vi "000_Project Manage.vi"(11 "Queue Ref In":T1={"UI"=refnum, "Message"=refnum, "Data"=refnum, "Caller"=refnum, "Name"="000 Common", "Data Path"=path "", "Class Path"=path "", "SubPanel"=refnum, "Project Name"="", "MNT"="", "Title"="", "Data Source"=refnum, "Queue List"={}, "VI"=refnum, "UE"=refnum}) -> ()   [LabVIEW 2020]
doc: "PM"
uses:
  Alin/QMH/000 Module Data Type.ctl
  Alin/QMH/Queue Message.ctl
  9999 SubVI/Global/Data Global/Data Global Mode.ctl
  ed3733e6-0b6c-4e46-af2e-562a3ca12228.vi
  <vilib>/Utility/file.llb/Read Delimited Spreadsheet (string).vi
  006 Path Management/006 System Gloabl.vi
  <vilib>/zip/NI_Unzip.lvlib
panel:
  in  "Project Refresh":bool
  in  "Monitor":bool
  in  "Project Set":bool
  in  "Project Copy":bool
  in  "Project Export":bool
  in  "Project Import":bool
  in  "Project Launch":bool
  in  "Project Delete":bool
  in  "Project List":i32(listbox)
  in  "Panel Hidden":bool
  in  "Data Source List":string(tree)
  out "Count":string
  in  "Device List":i32(listbox)
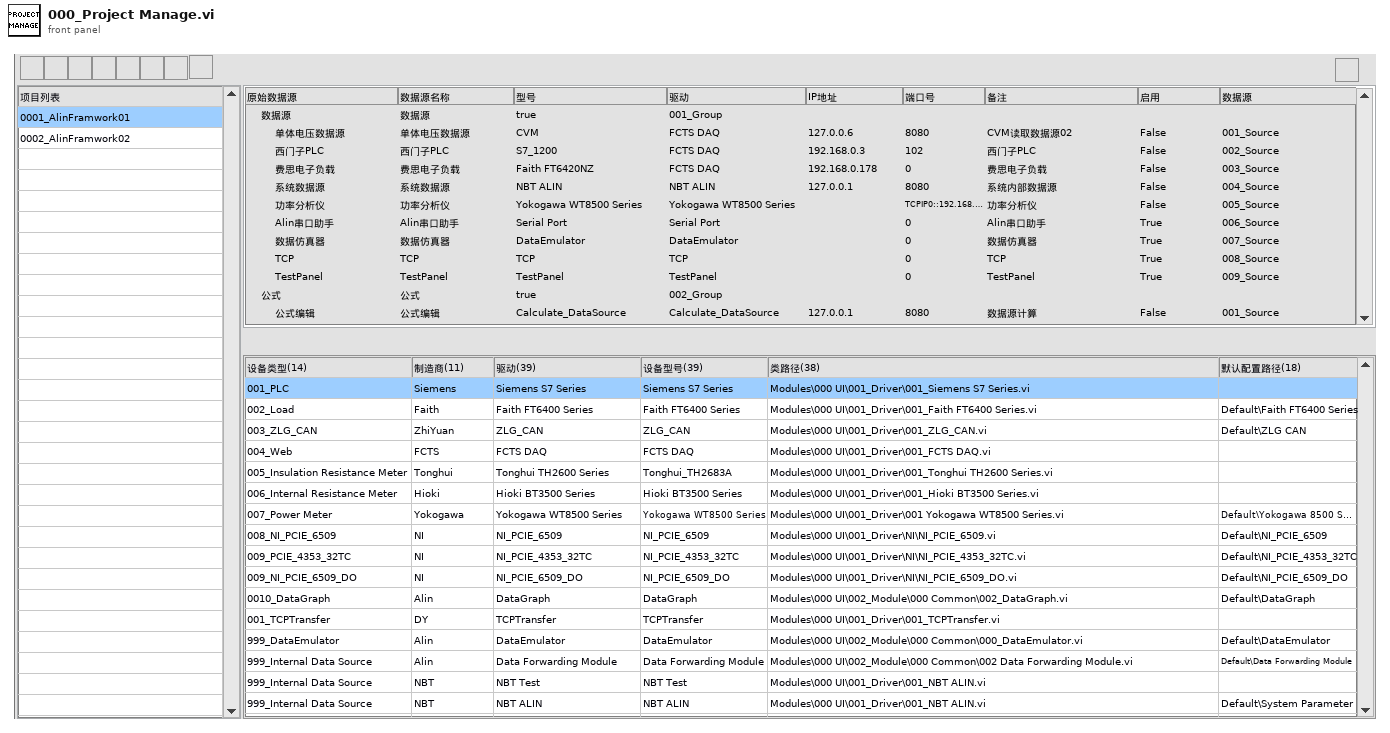
[diagram p1: front panel]
types:
  T1 = typedef "000 Module Data Type.ctl" = cluster{"UI":refnum<queue>, "Message":refnum<queue>, "Data":refnum<queue>, "Caller":refnum<queue>, "Name":string, "Data Path":path, "Class Path":path, "SubPanel":refnum<vi>, "Project Name":string, "MNT":string, "Title":string, "Data Source":refnum<queue>, "Queue List":map{string, refnum<queue>}, "VI":refnum<vi>, "UE":refnum<user-event>}
  T2 = cluster{"Project":string, "Queue List":map{string, refnum<queue>}, "Queue Ref":T1, "RootPath":path, "Device List Ref":refnum<vi>, "Config Path":path, "Project List Value":i32, "Project List":string[], "Project List Refer":refnum<vi>, "Source":refnum<vi>, "Source Path":path}
  T3 = cluster{"Read Data":map{string, string}, "Send Data":map{string, string}, "Open?":bool, "Start?":bool, "Queue Ref":T1, "Device List":refnum<vi>}
  T4 = enum32{"Invalid", "Standard", "Closed", "Hidden", "Minimized", "Maximized"}
  T5 = typedef "eventvkey.ctl" = enum16{"ASCII", "Enter", "Return", "Shift", "Ctrl", "Alt", "Cmd", "Opt", "Caps", "NumLock", "Clear", "Break", "Up", "Down", "Left", "Right", "Insert", "Delete", "Home", "End", "PageUp", "PageDown", "Escape", "Help", "Pause", "ScrollLock", "F1", "F2", "F3", "F4", "F5", "F6", "F7", "F8", "F9", "F10", "F11", "F12", "F13", "F14", "F15", "F16", "F17", "F18", "F19", "F20", "F21", "F22", "F23", "F24", "Play", "VolumeUp", "VolumeDown", "Mute", "Two Byte Char"}
  T6 = cluster{"Shift":bool, "Ctrl":bool, "Alt":bool, "Cmd":bool, "Opt":bool}
  T7 = typedef "Data Global Mode.ctl" = enum16{"Init", "Read", "Write", "Write Data", "Load"}
  T8 = enum32{"invalid app kind", "Development System", "Run Time System", "Student Edition", "Embedded LabVIEW", "Evaluation", "Custom"}
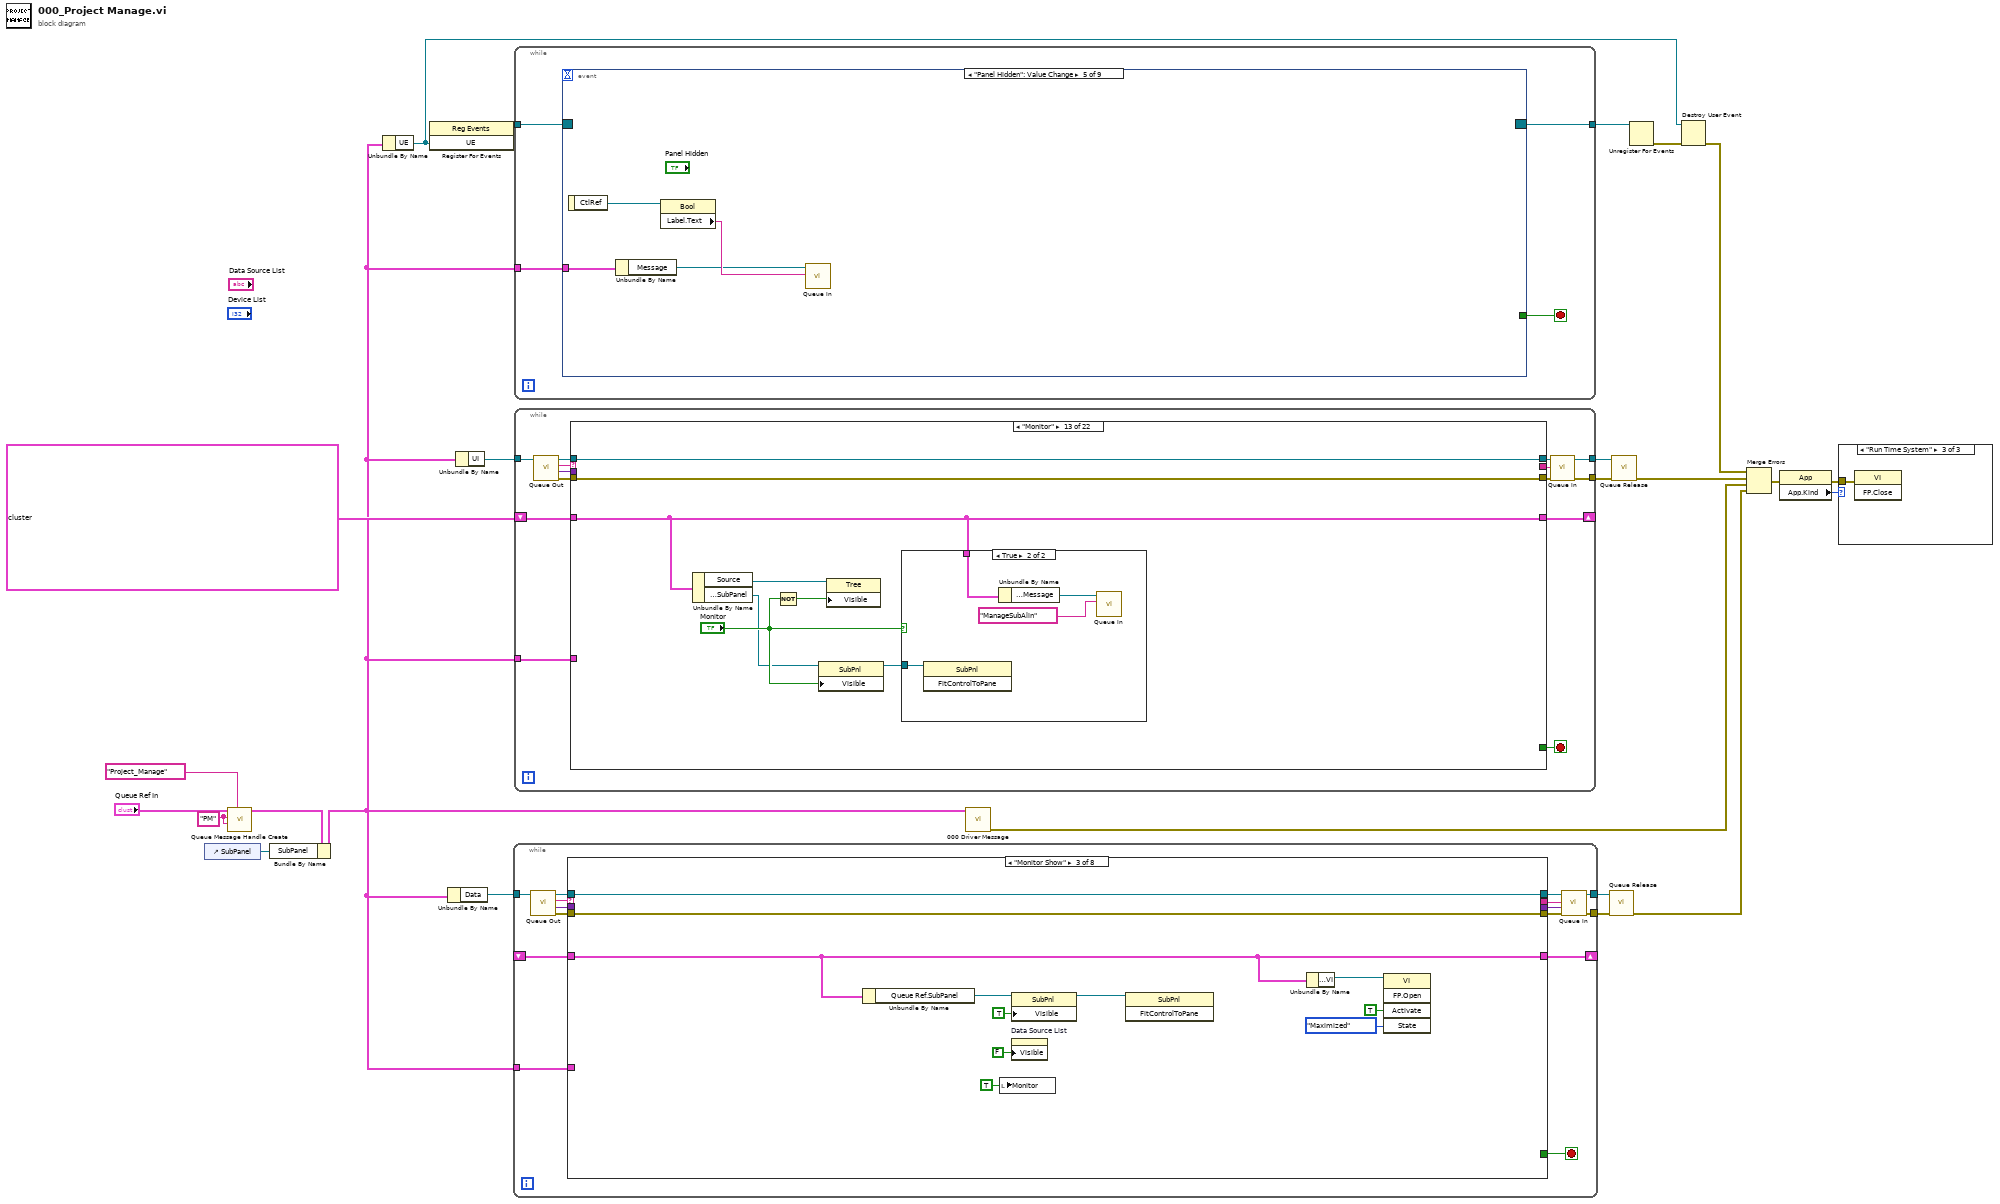
[diagram p0: block diagram]
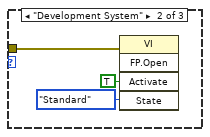
[diagram p3: hidden frame]
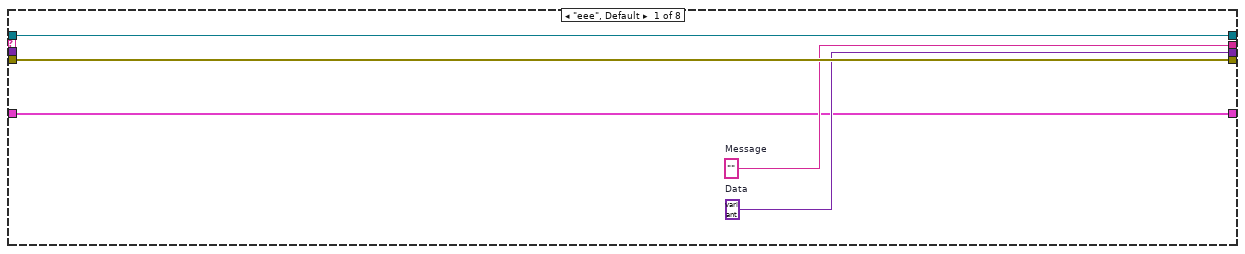
[diagram p4: hidden frame]
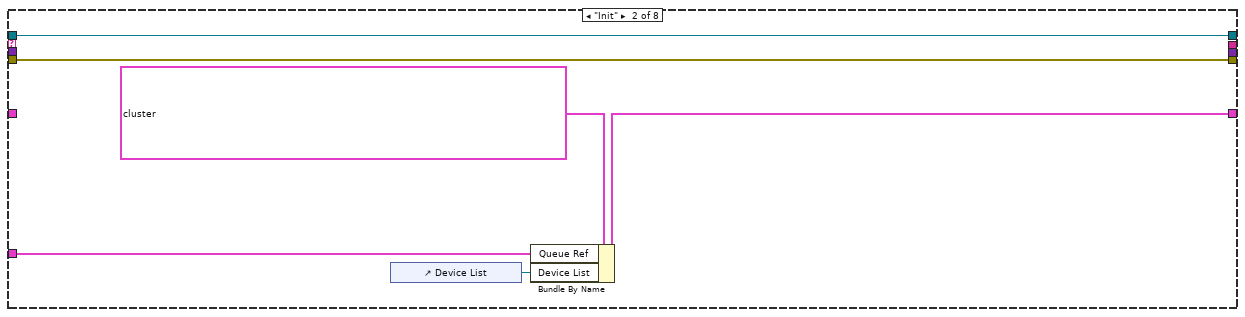
[diagram p5: hidden frame]
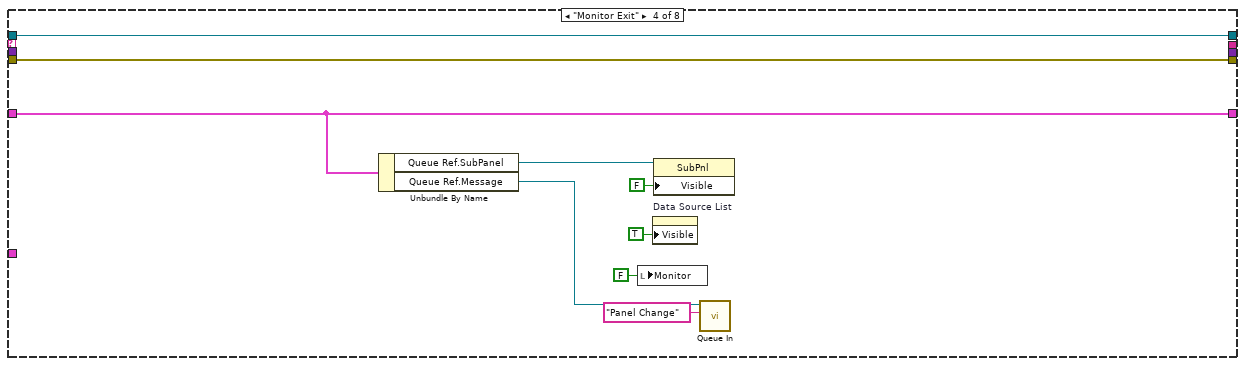
[diagram p6: hidden frame]
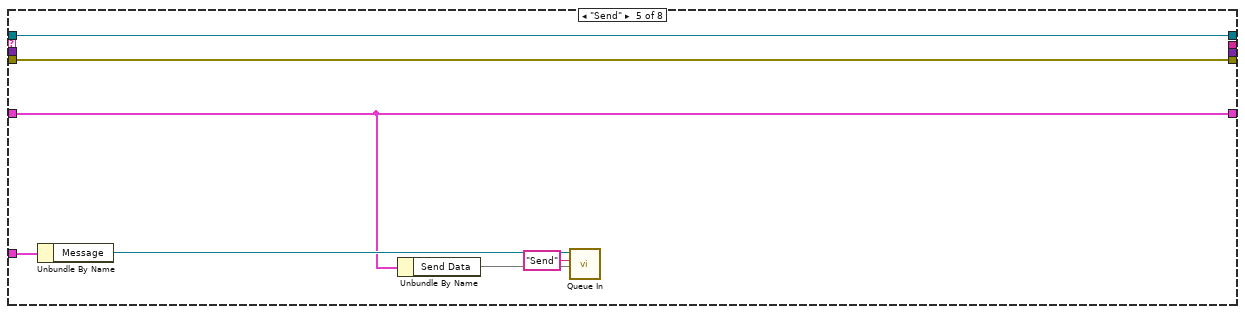
[diagram p7: hidden frame]
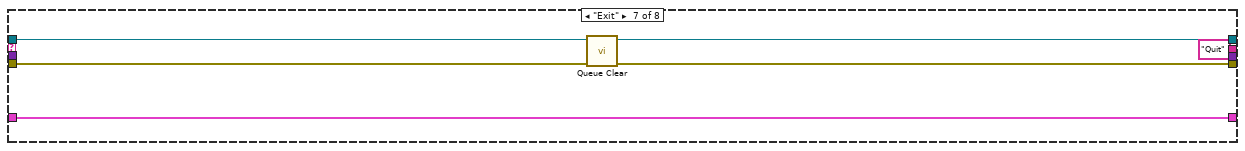
[diagram p9: hidden frame]
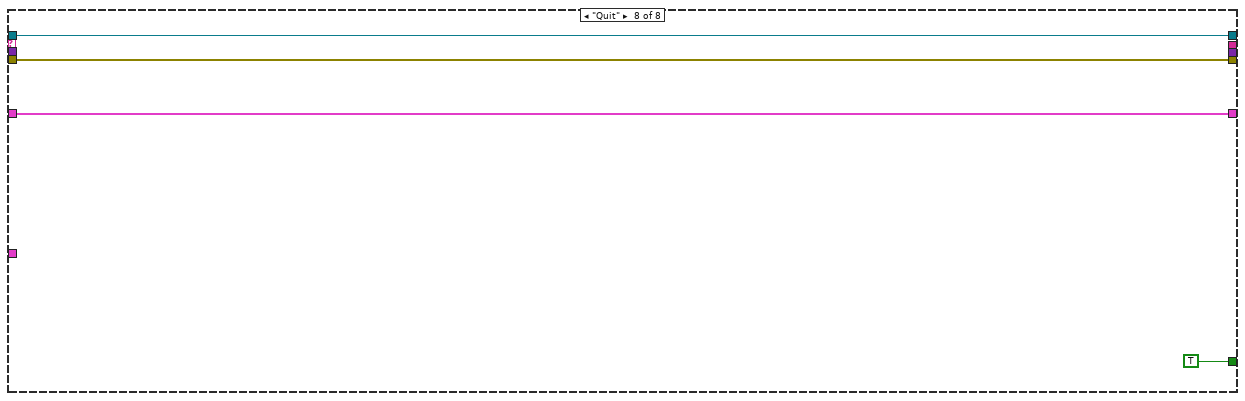
[diagram p10: hidden frame]
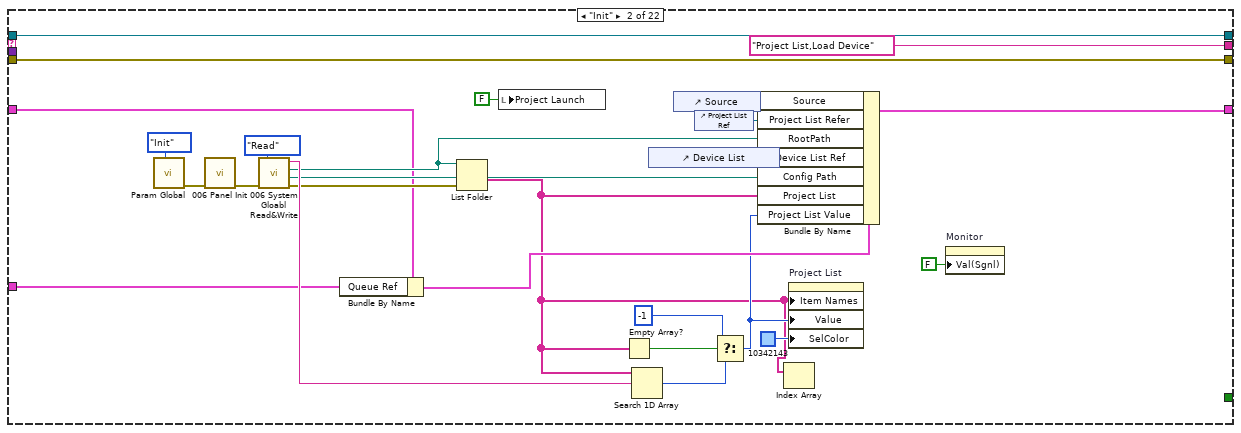
[diagram p12: hidden frame]
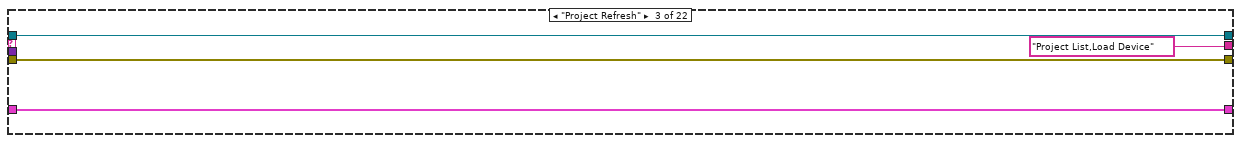
[diagram p13: hidden frame]
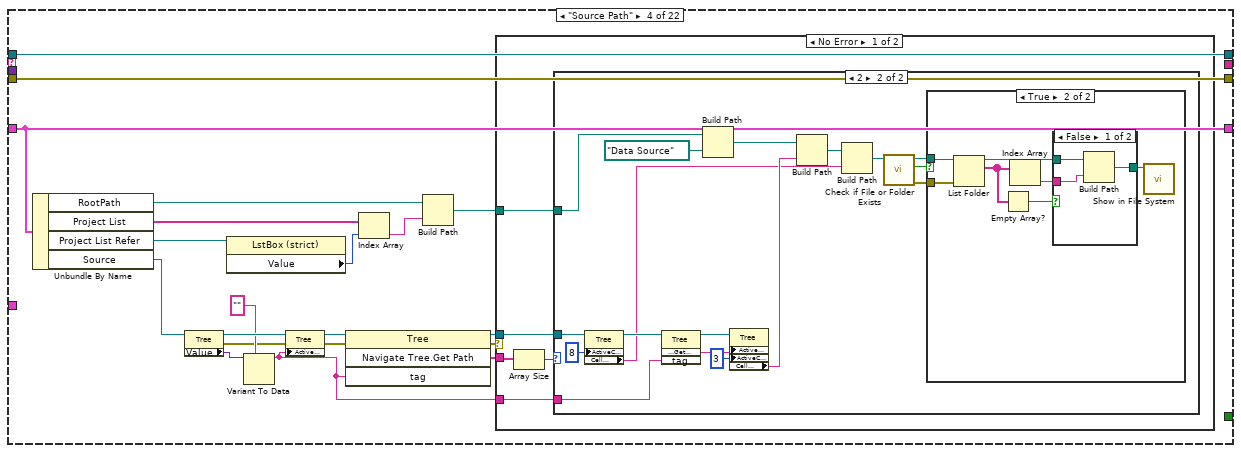
[diagram p14: hidden frame]
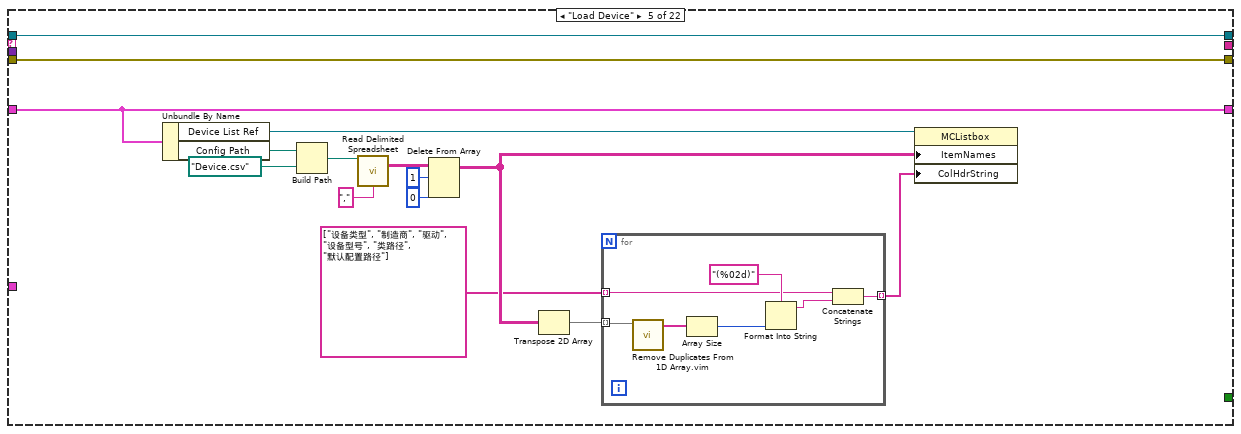
[diagram p19: hidden frame]
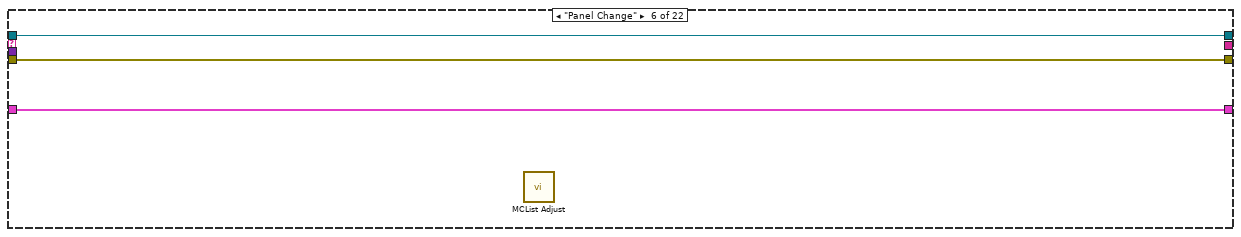
[diagram p20: hidden frame]
diagram:
  w4 = "PM" ("Title")
  n1 = control-ref of="SubPanel"() -> (w1:refnum<vi>)
  n2 = call "Queue Message Handle Create.vi"("Project Name"="Project_Manage" ("Name"), "Name"=w4, "Title"=w4, "Queue Ref In"="Queue Ref In") -> ("Queue Ref Out"=w9:T1)  [unwired: 6 in, 1 out]
  n3 = Bundle By Name(cluster=w9, "SubPanel"=w1) -> (w2:T1)
  n4 = Unbundle By Name(w2) -> ("UE"=w8:refnum<user-event>)
  n5 = register-events(w8) -> (reference out=w12:refnum<event-registration>)  [unwired: 2 in, 1 out]
  n6 = Unbundle By Name(w2) -> ("Data"=w22:refnum<queue>)
  n7 = Unbundle By Name(w2) -> ("UI"=w17:refnum<queue>)
  n8 = while {
    tunnel: w22 -> [w35]
    tunnel: [w32] -> w20
    tunnel: [w31] -> w21
    shift-right: [w27] -> _
    shift-left: _ -> [w26]
    tunnel: w2 -> [w25]
    stop <- w39 stop-if-true
    n9 = call "Queue Out.vi"("Queue In"=w35) -> ("error out"=w38:errorcluster, "Data"=w36:variant, "Message"=w37:string, "Queue Out"=w34:refnum<queue>)  [unwired: 6 in, 1 out]
    n10 = case shown="\"Monitor Show\"" w37 {
      tunnel: w34 -> [w44 w50 w61 w70 w77 w80 w85 w89]
      tunnel: w38 -> [w43 w49 w60 w69 w76 w79 w83 w90]
      tunnel: [w44 w50 w61 w70 w77 w80 w84 w89] -> w33
      tunnel: [w43 w49 w60 w69 w76 w79 w82 w90] -> w30
      tunnel: [w42 _ _ _ _ _ "Quit" _] -> w29
      tunnel: [_ _ _ _ _ _ _ TRUE] -> w39
      tunnel: [w41 _ _ _ _ _ _ _] -> w28
      tunnel: w36 -> [_ _ _ _ _ _ _ _]
      tunnel: [w40 w47 w54 w68 w73 w78 w81 w87] -> w27
      tunnel: w26 -> [w40 _ w54 w68 w73 w78 w81 w87]
      tunnel: w25 -> [_ w46 _ _ w75 _ _ _]
      frame "eee", Default {
        w41 = variant  # Data
        w42 = ""  # Message
      }
      frame "Init" {
        n11 = control-ref of="Device List"() -> (w45:refnum<vi>)
        n12 = Bundle By Name(cluster=T3 {"Read Data"={}, "Send Data"={}, "Open?"=FALSE, "Start?"=FALSE, "Queue Ref"={"UI"=refnum, "Message"=refnum, "Data"=refnum, "Caller"=refnum, "Name"="", "Data Path"=path "", "Class Path"=path "", "SubPanel"=refnum, "Project Name"="", "MNT"="", "Title"="", "Data Source"=refnum, "Queue List"={}, "VI"=refnum, "UE"=refnum}, "Device List"=refnum}, "Queue Ref"=w46, "Device List"=w45) -> (w47:T3)
      }
      frame "Monitor Show" {
        n13 = Unbundle By Name(w54) -> ("Queue Ref.SubPanel"=w59:refnum<vi>)
        n14 = local write "Monitor"(TRUE ("Monitor")) -> ()
        n15 = property on="Data Source List" class="Tree (严格)"("Visible"=FALSE ("可见")) -> ()  [unwired: 2 in, 2 out]
        n16 = property class="SubPnl"(reference=w59, "Visible"=TRUE ("可见")) -> (reference out=w56:refnum<vi>)  [unwired: 1 in, 1 out]
        n17 = invoke class="SubPnl" method="FitControlToPane"(reference=w56) -> ()  [unwired: 2 in, 3 out]
        n18 = Unbundle By Name(w54) -> ("Queue Ref.VI"=w53:refnum<vi>)
        n19 = invoke class="VI" method="FP.Open"(reference=w53, "Activate"=TRUE ("激活？"), "State"=T4."Maximized" ("状态")) -> ()  [unwired: 2 in, 5 out]
      }
      frame "Monitor Exit" {
        n20 = Unbundle By Name(w68) -> ("Queue Ref.SubPanel"=w67:refnum<vi>, "Queue Ref.Message"=w63:refnum<queue>)
        n21 = local write "Monitor"(FALSE ("Monitor")) -> ()
        n22 = property on="Data Source List" class="Tree (严格)"("Visible"=TRUE ("可见")) -> ()  [unwired: 2 in, 2 out]
        n23 = property class="SubPnl"(reference=w67, "Visible"=FALSE ("可见")) -> ()  [unwired: 1 in, 2 out]
        n24 = call "Queue In.vi"("Message"="Panel Change", "Queue In"=w63) -> ()  [unwired: 8 in, 2 out]
      }
      frame "Send" {
        n25 = Unbundle By Name(w75) -> ("Message"=w74:refnum<queue>)
        n26 = Unbundle By Name(w73) -> ("Send Data"=w72:map{string, string})
        n27 = call "Queue In.vi"("Data"=w72, "Message"="Send", "Queue In"=w74) -> ()  [unwired: 7 in, 2 out]
      }
      frame "Read" {
      }
      frame "Exit" {
        n28 = call "Queue Clear.vi"("error in (no error)"=w83, "Queue In"=w85) -> ("error out"=w82:errorcluster, "Queue Out"=w84:refnum<queue>)  [unwired: 8 in]
      }
      frame "Quit" {
      }
    }
    n29 = call "Queue In.vi"("error in (no error)"=w30, "Data"=w28, "Message"=w29, "Queue In"=w33) -> ("error out"=w31:errorcluster, "Queue Out"=w32:refnum<queue>)  [unwired: 6 in]
  }
  n30 = while {
    tunnel: w12 -> [w94]
    tunnel: [w92] -> w13
    tunnel: w2 -> [w91]
    stop <- w93 stop-if-true
    n31 = event shown="[4] \"Panel Hidden\": Value Change" {
      selector: w94 -> [_ _ _ _ _ _ _ _ _]
      dyn-events: [_ _ _ _ _ _ _ _ _] -> w92
      timeout: _ -> [_ _ _ _ _ _ _ _ _]
      tunnel: [_ _ _ _ _ _ _ w119 _] -> w93
      tunnel: w91 -> [_ w95 w102 w105 w109 w113 w116 _ w123]
      event Timeout {
        n32 = event-data() -> ()  [unwired: 1 in, 1 out]
      }
      event Key Down {
        n33 = event-data() -> ("Char"=w99:i16, "VKey"=w98:T5, "Mods"=w97:cluster{"Num Pad":bool, "Menu Key":bool}, "PlatMods"=w96:T6)  [unwired: 1 in]
        n34 = call "Queue Key Down.vi"("Queue Ref Out"=w95, "C"=w99, "Platform Key"=w96, "Group Key"=w97, "V Key"=w98) -> ()  [unwired: 6 in, 1 out]
      }
      event Panel Resize {
        n35 = event-data() -> ()  [unwired: 1 in, 1 out]
        n36 = Unbundle By Name(w102) -> ("Message"=w101:refnum<queue>)
        n37 = call "Queue In.vi"("Message"="Panel Change", "Queue In"=w101) -> ()  [unwired: 8 in, 2 out]
      }
      event "Project Delete", "Project Launch", "Project List", "Project Import", "Project Export", "Project Copy", "Project Set", "Monitor", "Project Refresh": Value Change {
        n38 = event-data() -> ("CtlRef"=w106:refnum<vi>)  [unwired: 1 in]
        n39 = Unbundle By Name(w105) -> ("UI"=w104:refnum<queue>)
        n40 = property class="Ctl"(reference=w106) -> ("Label.Text"=w103:string)  [unwired: 1 in, 2 out]
        n41 = call "Queue In.vi"("Message"=w103, "Queue In"=w104) -> ()  [unwired: 8 in, 2 out]
      }
      event "Panel Hidden": Value Change {
        n42 = event-data() -> ("CtlRef"=w110:refnum<vi>)  [unwired: 1 in]
        n43 = Unbundle By Name(w109) -> ("Message"=w107:refnum<queue>)
        n44 = property class="Bool"(reference=w110) -> ("Label.Text"=w108:string)  [unwired: 1 in, 2 out]
        n45 = call "Queue In.vi"("Message"=w108, "Queue In"=w107) -> ()  [unwired: 8 in, 2 out]
      }
      event "Data Source List": Double Click {
        n46 = event-data() -> ()  [unwired: 1 in, 1 out]
        n47 = Unbundle By Name(w113) -> ("UI"=w112:refnum<queue>)
        n48 = call "Queue In.vi"("Message"="Source Path", "Queue In"=w112) -> ()  [unwired: 8 in, 2 out]
      }
      event "Project List": Double Click {
        n49 = event-data() -> ("PlatMods.Ctrl"=w114:bool)  [unwired: 1 in]
        n50 = Unbundle By Name(w116) -> ("UI"=w115:refnum<queue>)
        n51 = case shown="True" w114 {
          tunnel: w115 -> [_ w118]
          frame False {
          }
          frame True {
            n52 = call "Queue In.vi"("Message"="Panel Show", "Queue In"=w118) -> ()  [unwired: 8 in, 2 out]
          }
        }
      }
      event User Event {
        n53 = event-data() -> ("Message"=w121:string)  [unwired: 1 in]
        n54 = Equal?(x=w121, y="Exit") -> (x = y?=w119:bool)
      }
      event Panel Close? {
        n55 = event-data() -> ()  [unwired: 1 in, 1 out]
        n56 = Unbundle By Name(w123) -> ("Message"=w122:refnum<queue>)
        n57 = Call Chain() -> (call chain=w126:string[])
        n58 = Array Size(array=w126) -> (size(s)=w125:i32)
        n59 = case shown="2.." w125 {
          tunnel: ["Exit Prepare" ("Message") "Panel Hidden" ("Message")] -> w124
          frame 0, Default {
          }
          frame 2.. {
          }
        }
        n60 = call "Queue In.vi"("Message"=w124, "Queue In"=w122) -> ()  [unwired: 8 in, 2 out]
        n61 = event-data("Discard?"=TRUE ("放弃？")) -> ()  [unwired: 1 in, 1 out]
      }
    }
  }
  n62 = while {
    tunnel: w17 -> [w139]
    tunnel: [w136] -> w15
    tunnel: [w135] -> w16
    tunnel: w2 -> [w132]
    shift-right: [w131] -> _
    shift-left: T2 {"Project"="", "Queue List"={}, "Queue Ref"={"UI"=refnum, "Message"=refnum, "Data"=refnum, "Caller"=refnum, "Name"="", "Data Path"=path "", "Class Path"=path "", "SubPanel"=refnum, "Project Name"="", "MNT"="", "Title"="", "Data Source"=refnum, "Queue List"={}, "VI"=refnum, "UE"=refnum}, "RootPath"=path "", "Device List Ref"=refnum, "Config Path"=path "", "Project List Value"=0, "Project List"=[], "Project List Refer"=refnum, "Source"=refnum, "Source Path"=path ""} -> [w130]
    stop <- w143 stop-if-true
    n63 = call "Queue Out.vi"("Queue In"=w139) -> ("error out"=w142:errorcluster, "Data"=w140:variant, "Message"=w141:string, "Queue Out"=w138:refnum<queue>)  [unwired: 6 in, 1 out]
    n64 = case shown="\"Monitor\"" w141 {
      selector: w141 -> [_ _ _ _ _ _ _ _ _ _ _ _ _ _ _ _ _ w488 _ _ _ _]
      tunnel: w138 -> [w146 w172 w176 w196 w244 w254 w270 w275 w312 w363 w394 w437 w462 w472 w481 w484 w487 w494 w497 w502 w510 w514]
      tunnel: w142 -> [w145 w171 w175 w195 w243 w253 w269 w277 w311 w362 w393 w436 w461 w471 w480 w483 w486 w493 w496 w501 w508 w515]
      tunnel: [w146 w172 w176 w196 w244 w254 w270 w275 w312 w363 w394 w437 w462 w472 w481 w484 w487 w494 w497 w502 w509 w514] -> w137
      tunnel: [w145 w171 w175 w195 w243 w253 w269 w277 w311 w362 w393 w436 w461 w471 w480 w483 w486 w493 w496 w501 w507 w515] -> w134
      tunnel: [_ "Project List,Load Device" ("Message") "Project List,Load Device" ("Message") _ _ _ _ _ _ _ _ "Project Tree" ("Message") _ _ "Load Project Info" ("Message") _ _ _ _ _ "Quit" _] -> w133
      tunnel: [_ _ _ _ _ _ _ _ _ _ _ _ _ _ _ _ _ _ _ _ _ TRUE] -> w143
      tunnel: w140 -> [_ _ _ _ _ _ _ _ _ _ _ _ _ _ _ _ _ _ _ w498 _ _]
      tunnel: w132 -> [_ w163 _ _ _ _ _ _ _ _ _ _ _ _ _ _ _ _ _ _ _ _]
      tunnel: [w144 w160 w174 w194 w238 w252 w258 w276 w296 w361 w387 w435 w459 w470 w479 w482 w485 w492 w495 w499 w506 w512] -> w131
      tunnel: w130 -> [w144 w155 w174 w194 w238 w252 w261 w276 w298 w361 w388 w434 w459 w470 w474 w482 w485 w492 w495 w500 w506 w512]
      frame "eee", Default {
      }
      frame "Init" {
        n65 = call "Param Global.vi"("Operate"=Data_Global_Mode."Init") -> ("error out"=w152:errorcluster)  [unwired: 9 in, 1 out]
        n66 = call "006 Panel Init.vi"("error in (no error)"=w152) -> ("error out"=w151:errorcluster)  [unwired: 10 in]
        n67 = call "006 System Gloabl Read&Write.vi"("error in (no error)"=w151, "RW"=enum16{"Read", "Write"}."Read") -> ("error out"=w161:errorcluster, "Config Path"=w157:path, "Root Path"=w159:path, "Project"=w168:string)  [unwired: 6 in]
        n68 = Bundle By Name(cluster=w155, "Queue Ref"=w163) -> (w164:T2)
        n69 = List Folder(path=w159, error in=w161) -> (folder names=w148:string[])  [unwired: 2 in, 3 out]
        n70 = local write "Project Launch"(FALSE ("Project Launch")) -> ()
        n71 = Empty Array?(array=w148) -> (empty?=w170:bool)
        n72 = Search 1D Array(1D array=w148, element=w168) -> (index of element=w167:i32)  [unwired: 1 in]
        n73 = control-ref of="Device List"() -> (w158:refnum<vi>)
        n74 = control-ref of="Source"() -> (w150:refnum<vi>)
        n75 = control-ref of="Project List Ref"() -> (w156:refnum<vi>)
        n76 = Select(t=-1 ("Project List"), s=w170, f=w167) -> (s? t:f=w149:i32)
        n77 = Bundle By Name(cluster=w164, "Source"=w150, "Project List Refer"=w156, "RootPath"=w159, "Device List Ref"=w158, "Config Path"=w157, "Project List"=w148, "Project List Value"=w149) -> (w160:T2)
        n78 = Index Array(array=w148) -> ()  [unwired: 1 in, 1 out]
        n79 = property on="Project List" class="LstBox (严格)"("Item Names"=w148, "Value"=w149, "SelColor"=u32 10342143 ("选择颜色")) -> ()  [unwired: 2 in, 2 out]
        n80 = property on="Monitor" class="Bool (严格)"("Val(Sgnl)"=FALSE ("值(信号)")) -> ()  [unwired: 2 in, 2 out]
      }
      frame "Project Refresh" {
      }
      frame "Source Path" {
        n81 = Unbundle By Name(w194) -> ("RootPath"=w193:path, "Project List"=w191:string[], "Project List Refer"=w192:refnum<vi>, "Source"=w186:refnum<vi>)
        n82 = property class="Tree"(reference=w186) -> (reference out=w188:refnum<vi>, error out=w179:errorcluster, "Value"=w187:variant)  [unwired: 1 in]
        n83 = property class="LstBox (strict)"(reference=w192) -> ("Value"=w190:i32)  [unwired: 1 in, 2 out]
        n84 = Variant To Data(type="", Variant=w187) -> (data=w177:string)  [unwired: 1 in, 1 out]
        n85 = property class="Tree"(reference=w188, error in=w179, "Active Item Tag"=w177) -> (reference out=w180:refnum<vi>, error out=w178:errorcluster)
        n86 = invoke class="Tree" method="Navigate Tree.Get Path"(reference=w180, error in=w178, "tag"=w177) -> (reference out=w182:refnum<vi>, error out=w184:errorcluster, "Navigate Tree:Get Path"=w183:string[])  [unwired: 1 in, 1 out]
        n87 = Index Array(array=w191, index=w190) -> (element=w189:string)
        n88 = Build Path(base path=w193, name or relative path=w189) -> (appended path=w181:path)
        n89 = case shown="No Error" w184 {
          tunnel: w183 -> [w201 _]
          tunnel: w182 -> [w199 _]
          tunnel: w181 -> [w198 _]
          tunnel: w177 -> [w197 _]
          frame No Error {
            n90 = Array Size(array=w201) -> (size(s)=w200:i32)
            n91 = case shown="2" w200 {
              tunnel: w199 -> [_ w217]
              tunnel: w198 -> [_ w204]
              tunnel: w197 -> [_ w215]
              frame 0, Default {
              }
              frame 2 {
                n92 = property class="Tree"(reference=w217, "ActiveColNum"=8 ("活动单元格:活动列数")) -> (reference out=w216:refnum<vi>, "Cell String"=w209:string)  [unwired: 1 in, 1 out]
                n93 = invoke class="Tree" method="Navigate Tree.Get Parent"(reference=w216, "tag"=w215) -> (reference out=w213:refnum<vi>, "Navigate Tree:Get Parent"=w212:string)  [unwired: 2 in, 2 out]
                n94 = Build Path(base path=w204, name or relative path=path "Data Source" ("名称或相对路径")) -> (appended path=w202:path)
                n95 = property class="Tree"(reference=w213, "Active Item Tag"=w212, "ActiveColNum"=3 ("活动单元格:活动列数")) -> ("Cell String"=w211:string)  [unwired: 1 in, 2 out]
                n96 = Build Path(base path=w202, name or relative path=w211) -> (appended path=w210:path)
                n97 = Build Path(base path=w210, name or relative path=w209) -> (appended path=w205:path)
                n98 = call <vilib>:"Check if File or Folder Exists.vi"("path"=w205) -> ("error out"=w207:errorcluster, "file or folder exists?"=w208:bool, "dup path"=w206:path)  [unwired: 8 in]
                n99 = case shown="True" w208 {
                  tunnel: w206 -> [_ w225]
                  tunnel: w207 -> [_ w224]
                  frame False {
                  }
                  frame True {
                    n100 = List Folder(path=w225, error in=w224) -> (path out=w220:path, filenames=w222:string[])  [unwired: 2 in, 2 out]
                    n101 = Empty Array?(array=w222) -> (empty?=w223:bool)
                    n102 = Index Array(array=w222) -> (element=w221:string)  [unwired: 1 in]
                    n103 = case shown="False" w223 {
                      tunnel: w221 -> [w227 _]
                      tunnel: w220 -> [w228 w229]
                      tunnel: [w226 w229] -> w219
                      frame False {
                        n104 = Build Path(base path=w228, name or relative path=w227) -> (appended path=w226:path)
                      }
                      frame True {
                      }
                    }
                    n105 = call <vilib>:"Show in File System.vi"("file or directory path"=w219) -> ()  [unwired: 10 in, 1 out]
                  }
                }
              }
            }
          }
          frame Error {
          }
        }
      }
      frame "Load Device" {
        n106 = Unbundle By Name(w238) -> ("Device List Ref"=w237:refnum<vi>, "Config Path"=w235:path)
        n107 = Build Path(base path=w235, name or relative path=path "Device.csv" ("名称或相对路径")) -> (appended path=w242:path)
        n108 = call-poly <vilib>:"Read Delimited Spreadsheet.vi"("file path (dialog if empty)"=w242, "delimiter (\\t)"="," ("delimiter (\\t)")) -> ("all rows"=w240:string[][])  [unwired: 8 in, 5 out]
        n109 = Delete From Array(array=w240, length=1 ("长度"), index (row)=0 ("索引 (行)")) -> (array with subset deleted=w233:string[][])  [unwired: 1 in, 1 out]
        n110 = Transpose 2D Array(2D array=w233) -> (transposed array=w232:string[][])
        n111 = for {
          tunnel: w232 -> [w251] mode=indexing
          tunnel: string[] ["设备类型", "制造商", "驱动", "设备型号", "类路径", "默认配置路径"] -> [w247] mode=indexing
          tunnel: [w245] -> w230 mode=indexing
          n112 = call "Remove Duplicates From 1D Array.vim"("array"=w251) -> ("array with duplicates removed"=w250:string[])  [unwired: 10 in]
          n113 = Array Size(array=w250) -> (size(s)=w248:i32)
          n114 = Format Into String(format string="(%02d)" ("格式字符串"), w248) -> (resulting string=w246:string)  [unwired: 2 in, 1 out]
          n115 = Concatenate Strings(w247, w246) -> (w245:string)
        }
        n116 = property class="MCListbox"(reference=w237, "ItemNames"=w233, "ColHdrString"=w230) -> ()  [unwired: 1 in, 2 out]
      }
      frame "Panel Change" {
        n117 = call "MCList Adjust.vi"() -> ()  [unwired: 11 in, 1 out]
      }
      frame "Project Delete" {
        n118 = Unbundle By Name(w261) -> ("RootPath"=w266:path, "Project List"=w268:string[], "Project List Value"=w267:i32)
        n119 = Index Array(array=w268, index=w267) -> (element=w265:string)
        n120 = Two Button Dialog(message="确定要删除项目吗？" ("消息")) -> (T button?=w262:bool)  [unwired: 2 in]
        n121 = Build Path(base path=w266, name or relative path=w265) -> (appended path=w264:path)
        n122 = case shown="True" w262 {
          tunnel: w264 -> [_ w273]
          tunnel: [_ w271] -> w256
          frame False {
          }
          frame True {
            n123 = Delete(path (use dialog)=w273, entire hierarchy (F)=TRUE ("整个层次结构(F)")) -> (error out=w271:errorcluster)  [unwired: 3 in, 2 out]
          }
        }
        n124 = call <vilib>:"Clear Errors.vi"("error in (no error)"=w256) -> ("error out"=w255:errorcluster)  [unwired: 5 in, 1 out]
        n125 = Unbundle By Name(w261) -> ("Project List Refer"=w259:refnum<vi>, "RootPath"=w260:path)
        n126 = List Folder(path=w260, error in=w255) -> (folder names=w257:string[])  [unwired: 2 in, 3 out]
        n127 = property class="LstBox (strict)"(reference=w259, "Item Names"=w257) -> ()  [unwired: 1 in, 2 out]
        n128 = Bundle By Name(cluster=w261, "Project List"=w257) -> (w258:T2)
      }
      frame "Project Launch" {
        n129 = case shown="True" "Project Launch" {
          tunnel: w276 -> [w282 w285]
          frame False {
            n130 = Unbundle By Name(w282) -> ("Queue List"=w281:map{string, refnum<queue>}, "Project"=w280:string)
            n131 = Look In Map(map=w281, key=w280) -> (value=w279:refnum<queue>)  [unwired: 1 in, 1 out]
            n132 = call "Queue In.vi"("Message"="Exit Prepare", "Queue In"=w279) -> ()  [unwired: 8 in, 2 out]
          }
          frame True {
            n133 = vi-ref "002_NBT Testplatform V3.1.vi"() -> (w290:refnum<vi>)
            n134 = property class="VI"(reference=w290) -> ("Path"=w289:path)  [unwired: 1 in, 2 out]
            n135 = Unbundle By Name(w285) -> ("Queue Ref"=w292:T1, "Project"=w287:string)
            n136 = Unbundle By Name(w285) -> ("RootPath"=w284:path)
            n137 = property class="VI"("FP.State"=T4."Hidden" ("前面板窗口:状态")) -> ()  [unwired: 2 in, 2 out]
            n138 = Build Path(base path=w284, name or relative path=w287) -> (appended path=w286:path)
            n139 = call "Create Folder.vi"("Path In"=w286) -> ("Path Out"=w288:path)  [unwired: 9 in, 1 out]
            n140 = flat-sequence {
              tunnel: w287 -> [w293]
              frame #0 {
                n141 = global write "006 System Gloabl.vi" "Project"(w293) -> ()
              }
              frame #1 {
                n142 = call "006 System Gloabl Read&Write.vi"("RW"=enum16{"Read", "Write"}."Write") -> ()  [unwired: 7 in, 4 out]
              }
            }
            n143 = Bundle By Name(cluster=w292, "Name"=w287, "Class Path"=w289, "Data Path"=w288, "Project Name"=w287) -> (w291:T1)
            n144 = call "000 Client Launch.vi"("Queue Ref"=w291) -> ()  [unwired: 10 in, 1 out]
          }
        }
      }
      frame "Project Copy" {
        n145 = Unbundle By Name(w298) -> ("Project List"=w303:string[], "RootPath"=w305:path, "Project List"=w308:string[], "Project List Value"=w307:i32)
        n146 = Index Array(array=w308, index=w307) -> (element=w306:string)
        n147 = case shown="Default" w306 {
          selector: w306 -> [w315 _]
          tunnel: [w318 _] -> w310
          tunnel: [w317 _] -> w309
          tunnel: w305 -> [w316 _]
          tunnel: [w314 _] -> w304
          tunnel: [w313 _] -> w302
          frame Default {
            n148 = Build Path(base path=w316, name or relative path=w315) -> (appended path=w314:path)
            n149 = call "Data Source Add Group.vi"() -> ("Name"=w313:string, "OK？"=w318:bool, "Data Out"=w317:string[])  [unwired: 9 in]
          }
          frame "" {
          }
        }
        n150 = case shown="True" w310 {
          tunnel: w309 -> [_ _]
          tunnel: w298 -> [w319 w325]
          tunnel: w304 -> [_ w323]
          tunnel: [w319 w324] -> w297
          tunnel: w303 -> [_ w322]
          tunnel: w302 -> [_ w321]
          tunnel: [_ w320] -> w295
          frame False {
          }
          frame True {
            n151 = Search 1D Array(1D array=w322, element=w321) -> (index of element=w327:i32)  [unwired: 1 in]
            n152 = Less Than 0?(x=w327) -> (x < 0?=w326:bool)
            n153 = case shown="True" w326 {
              tunnel: w321 -> [w329 w342]
              tunnel: w325 -> [w328 w344]
              tunnel: [w328 w344] -> w324
              tunnel: w323 -> [_ w341]
              tunnel: [_ w332] -> w320
              frame False {
                n154 = Format Into String(format string="项目\"%s\"已存在！" ("消息"), w329) -> (resulting string=w330:string)  [unwired: 2 in, 1 out]
                n155 = One Button Dialog(message=w330) -> ()  [unwired: 1 in, 1 out]
              }
              frame True {
                n156 = Unbundle By Name(w344) -> ("RootPath"=w343:path)
                n157 = Build Path(base path=w343, name or relative path=w342) -> (appended path=w340:path)
                n158 = List Folder(path=w341) -> (path out=w335:path, filenames=w336:string[], folder names=w337:string[])  [unwired: 3 in, 1 out]
                n159 = call <vilib>:"Check if File or Folder Exists.vi"("path"=w340) -> ("error out"=w338:errorcluster, "dup path"=w339:path)  [unwired: 8 in, 1 out]
                n160 = Build Array (concatenate)(w336, w337) -> (w334:string[])
                n161 = Create Folder(path (use dialog)=w339, error in=w338) -> (created path=w333:path)  [unwired: 1 in, 2 out]
                n162 = for {
                  tunnel: w335 -> [w349]
                  tunnel: w334 -> [w348] mode=indexing
                  tunnel: w333 -> [w347]
                  tunnel: [w345] -> w332
                  n163 = Build Path(base path=w349, name or relative path=w348) -> (appended path=w346:path)
                  n164 = Copy(10:w347, 11:w346) -> (0:w345:errorcluster)  [unwired: 3 in, 2 out]
                }
              }
            }
          }
        }
        n165 = Unbundle By Name(w298) -> ("Project List Refer"=w300:refnum<vi>, "RootPath"=w301:path)
        n166 = List Folder(path=w301, error in=w295) -> (folder names=w299:string[])  [unwired: 2 in, 3 out]
        n167 = property class="LstBox (严格)"(reference=w300, "Item Names"=w299) -> ()  [unwired: 1 in, 2 out]
        n168 = Bundle By Name(cluster=w297, "Project List"=w299) -> (w296:T2)
      }
      frame "Project Export" {
        n169 = Unbundle By Name(w361) -> ("RootPath"=w358:path, "Project List"=w360:string[], "Project List Value"=w359:i32)
        n170 = Index Array(array=w360, index=w359) -> (element=w353:string)
        n171 = Concatenate Strings(w353, ".zip" ("字符串")) -> (w351:string)
        n172 = Build Path(base path=w358, name or relative path=w353) -> (appended path=w357:path)
        n173 = call "文件对话框"("default name"=w351, "pattern (all files)"="*.zip") -> ("selected path"=w355:path, "cancelled"=w350:bool, "error out"=w356:errorcluster)  [unwired: 10 in, 1 out]
        n174 = case shown="False" w350 {
          tunnel: w357 -> [w366 _]
          tunnel: w356 -> [w365 _]
          tunnel: w355 -> [w364 _]
          frame False {
            n175 = case shown="No Error" w365 {
              tunnel: w366 -> [w369 _]
              tunnel: w364 -> [w368 _]
              tunnel: [w367 _] -> _
              frame No Error {
                n176 = Strip Path(path=w369) -> (stripped path=w370:path)  [unwired: 1 out]
                n177 = call <vilib>:"Recursive File List.vi"("Folder Path"=w369) -> ("error out"=w372:errorcluster, "All Files in Dir"=w371:path[])  [unwired: 6 in, 3 out]
                n178 = call <vilib>:"New Zip File.vi"("error in (no error)"=w372, "target"=w368) -> ("error out"=w375:errorcluster, "zip file out"=w376:i64)  [unwired: 1 in, 3 out]
                n179 = for {
                  tunnel: w371 -> [w381] mode=indexing
                  tunnel: w375 -> [w378]
                  tunnel: [w382] -> w374
                  shift-right: [w383] -> w373
                  shift-left: w376 -> [w384]
                  tunnel: w370 -> [w380]
                  stop <- w382 stop-if-true
                  n180 = call <vilib>:"Compare Two Paths.vi"("error in (no error)"=w378, "Path 2"=w381, "Path 1"=w380) -> ("error out"=w377:errorcluster, "Relative Path from 1 to 2"=w379:path)  [unwired: 5 in, 2 out]
                  n181 = call <vilib>:"Add File to Zip.vi"("error in (no error)"=w377, "destination path in zip"=w379, "source file path"=w381, "zip file in"=w384) -> ("error out"=w382:errorcluster, "zip file out"=w383:i64)  [unwired: 6 out]
                }
                n182 = call <vilib>:"Close Zip File.vi"("error in (no error)"=w374, "zip file in"=w373) -> ("error out"=w367:errorcluster)  [unwired: 1 in, 4 out]
              }
              frame Error {
              }
            }
          }
          frame True {
          }
        }
      }
      frame "Project Import" {
        n183 = call <vilib>:"Set Busy.vi"() -> ("error out"=w386:errorcluster)  [unwired: 10 in, 1 out]
        n184 = call "文件对话框2"("pattern (all files)"="*.zip") -> ("selected path"=w391:path, "exists"=w389:bool, "error out"=w390:errorcluster)  [unwired: 11 in, 1 out]
        n185 = case shown="No Error" w390 {
          tunnel: w391 -> [w400 _]
          tunnel: w389 -> [w399 _]
          tunnel: w388 -> [w398 w424]
          tunnel: [w397 w424] -> w387
          tunnel: w386 -> [w396 w423]
          tunnel: [w395 w423] -> w385
          frame No Error {
            n186 = case shown="True" w399 {
              tunnel: w400 -> [_ w412]
              tunnel: w398 -> [w402 w405]
              tunnel: [w402 w403] -> w397
              tunnel: w396 -> [w401 w406]
              tunnel: [w401 w406] -> w395
              frame False {
              }
              frame True {
                n187 = Unbundle By Name(w405) -> ("RootPath"=w409:path)
                n188 = call <vilib>:"Check if File or Folder Exists.vi"("path"=w409) -> ("error out"=w414:errorcluster, "file or folder exists?"=w416:bool, "dup path"=w415:path)  [unwired: 8 in]
                n189 = case shown="False" w416 {
                  tunnel: w415 -> [w420 w421]
                  tunnel: w414 -> [w419 w422]
                  tunnel: [w418 w422] -> w413
                  tunnel: [w417 w421] -> w411
                  frame False {
                    n190 = Create Folder(path (use dialog)=w420, error in=w419) -> (created path=w417:path, error out=w418:errorcluster)  [unwired: 1 in, 1 out]
                  }
                  frame True {
                  }
                }
                n191 = Unbundle By Name(w405) -> ("Project List Refer"=w410:refnum<vi>)
                n192 = call <vilib>:"Unzip.vi"("error in (no error)"=w413, "Target directory (same as Zip file if empty)"=w411, "Zip file"=w412) -> ("error out"=w408:errorcluster)  [unwired: 6 in, 2 out]
                n193 = call <vilib>:"Clear Errors.vi"("error in (no error)"=w408) -> ("error out"=w407:errorcluster)  [unwired: 5 in, 1 out]
                n194 = List Folder(path=w409, error in=w407) -> (folder names=w404:string[])  [unwired: 2 in, 3 out]
                n195 = property class="LstBox (strict)"(reference=w410, "Item Names"=w404) -> ()  [unwired: 1 in, 2 out]
                n196 = Bundle By Name(cluster=w405, "Project List"=w404) -> (w403:T2)
              }
            }
          }
          frame Error {
          }
        }
        n197 = call <vilib>:"Unset Busy.vi"("error in (no error)"=w385) -> ()  [unwired: 10 in, 1 out]
      }
      frame "Project List" {
        n198 = Unbundle By Name(w434) -> ("Project List"=w433:string[])
        n199 = case shown="0.." "Project List" {
          selector: "Project List" -> [_ w446]
          tunnel: w433 -> [_ w447]
          tunnel: [_ w443] -> w428
          tunnel: w434 -> [w438 w439]
          tunnel: [w438 w439] -> w430
          frame -1, Default {
          }
          frame 0.. {
            n200 = property class="App"() -> ("App.Kind"=w440:T8)  [unwired: 2 in, 2 out]
            n201 = case shown="\"Run Time System\"" w440 {
              frame "invalid app kind", Default {
              }
              frame "Development System" {
              }
              frame "Run Time System" {
                n202 = property on="Project Launch" class="Bool (严格)"("Val(Sgnl)"=TRUE ("值(信号)")) -> ()  [unwired: 2 in, 2 out]
              }
            }
            n203 = Index Array(array=w447, index=w446) -> (element=w443:string)
            n204 = Unbundle By Name(w439) -> ("Queue List"=w445:map{string, refnum<queue>})
            n205 = Look In Map(map=w445, key=w443) -> (key not found?=w444:bool, value=w441:refnum<queue>)  [unwired: 1 in]
            n206 = First Call?() -> (First Call?: T/F=w442:bool)
            n207 = case shown="False" w442 {
              tunnel: w444 -> [w454 _]
              tunnel: w441 -> [w453 _]
              frame False {
                n208 = Not A Number/Path/Refnum?(number/path/refnum=w453) -> (NaN/Path/Refnum?=w452:bool)
                n209 = Not(x=w454) -> (.not. x?=w451:bool)
                n210 = Not(x=w452) -> (.not. x?=w450:bool)
                n211 = And(x=w451, y=w450) -> (x .and. y?=w449:bool)
                n212 = local write "Project Launch"(w449) -> ()
              }
              frame True {
              }
            }
          }
        }
        n213 = Unbundle By Name(w430) -> ("RootPath"=w429:path)
        n214 = Build Path(base path=w429, name or relative path=w428) -> (appended path=w427:path)
        n215 = Build Path(base path=w427, name or relative path=path "Data Source" ("名称或相对路径")) -> (appended path=w425:path)
        n216 = Bundle By Name(cluster=w430, "Project"=w428, "Project List Value"="Project List", "Source Path"=w425) -> (w435:T2)
      }
      frame "Monitor" {
        n217 = Unbundle By Name(w459) -> ("Source"=w458:refnum<vi>, "Queue Ref.SubPanel"=w455:refnum<vi>)
        n218 = Not(x="Monitor") -> (.not. x?=w457:bool)
        n219 = property class="SubPnl"(reference=w455, "Visible"="Monitor") -> (reference out=w460:refnum<vi>)  [unwired: 1 in, 1 out]
        n220 = property class="Tree"(reference=w458, "Visible"=w457) -> ()  [unwired: 1 in, 2 out]
        n221 = case shown="True" "Monitor" {
          tunnel: w459 -> [_ w466]
          tunnel: w460 -> [_ w463]
          frame False {
          }
          frame True {
            n222 = invoke class="SubPnl" method="FitControlToPane"(reference=w463) -> ()  [unwired: 2 in, 3 out]
            n223 = Unbundle By Name(w466) -> ("Queue Ref.Message"=w465:refnum<queue>)
            n224 = call "Queue In.vi"("Message"="ManageSubAlin", "Queue In"=w465) -> ()  [unwired: 8 in, 2 out]
          }
        }
      }
      frame "Project Tree" {
        n225 = Unbundle By Name(w470) -> ("Source Path"=w468:path, "Source"=w469:refnum<vi>)
        n226 = call "Data Source Tree Refresh.vi"("Tree In"=w469, "Data Path"=w468) -> ("Count"=→"Count":string)  [unwired: 7 in, 2 out]
      }
      frame "Project List0" {
        n227 = Unbundle By Name(w474) -> ("Project List Refer"=w473:refnum<vi>)
        n228 = property on="属性节点" class="LstBox (strict)"(reference=w473) -> ("Item Names"=w478:string[], "Value"=w477:i32)  [unwired: 1 in, 2 out]
        n229 = Index Array(array=w478, index=w477) -> (element=w476:string)
        n230 = Bundle By Name(cluster=w474, "Project"=w476) -> (w479:T2)
      }
      frame "Load Project Info" {
      }
      frame "Project Config" {
      }
      frame "Panel Hidden", "Panel Insert", "Panel Show" {
        n231 = Unbundle By Name(w492) -> ("Queue List"=w491:map{string, refnum<queue>}, "Project"=w490:string)
        n232 = Look In Map(map=w491, key=w490) -> (value=w489:refnum<queue>)  [unwired: 1 in, 1 out]
        n233 = call "Queue In.vi"("Message"=w488, "Queue In"=w489) -> ()  [unwired: 8 in, 2 out]
      }
      frame "====Message====" {
      }
      frame "Send Client Refer" {
        n234 = in-place {
          in-place-border: w498 -> [w505]
          n235 = in-place-cluster #1(w500) -> ("Queue List"=w504:map{string, refnum<queue>})
          n236 = Variant To Data(type=w504, Variant=w505) -> (data=w503:map{string, refnum<queue>})  [unwired: 1 in, 1 out]
          n237 = in-place-cluster #1("Queue List"=w503) -> (w499:T2)
        }
      }
      frame "Exit" {
        n238 = call "Queue Clear.vi"("error in (no error)"=w508, "Queue In"=w510) -> ("error out"=w507:errorcluster, "Queue Out"=w509:refnum<queue>)  [unwired: 8 in]
      }
      frame "Quit" {
      }
    }
    n239 = call "Queue In.vi"("error in (no error)"=w134, "Message"=w133, "Queue In"=w137) -> ("error out"=w135:errorcluster, "Queue Out"=w136:refnum<queue>)  [unwired: 7 in]
  }
  n240 = call "000 Driver Message.vi"("Queue In"=w2) -> ("error out"=w23:errorcluster)  [unwired: 8 in, 2 out]
  n241 = call "Queue Release.vi"("error in (no error)"=w21, "Queue In"=w20) -> ("error out"=w24:errorcluster)  [unwired: 9 in]
  n242 = call "Queue Release.vi"("error in (no error)"=w16, "Queue In"=w15) -> ("error out"=w19:errorcluster)  [unwired: 9 in]
  n243 = Unregister For Events(event registration refnum=w13) -> (error out=w14:errorcluster)  [unwired: 1 in]
  n244 = Destroy User Event(user event=w8, error in=w14) -> (error out=w18:errorcluster)
  n245 = Merge Errors(w18, w19, w23, w24) -> (w7:errorcluster)
  n246 = property class="App"(error in=w7) -> (error out=w6:errorcluster, "App.Kind"=w10:T8)  [unwired: 1 in, 1 out]
  n247 = case shown="\"Run Time System\"" w10 {
    tunnel: w6 -> [_ w516 w519]
    frame "invalid app kind", Default {
    }
    frame "Development System" {
      n248 = invoke class="VI" method="FP.Open"(error in=w516, "Activate"=TRUE ("激活？"), "State"=T4."Standard" ("状态")) -> ()  [unwired: 2 in, 5 out]
    }
    frame "Run Time System" {
      n249 = invoke class="VI" method="FP.Close"(error in=w519) -> ()  [unwired: 2 in, 3 out]
    }
  }
